vi "CmdGenerate.vi"(1 "Control Value":sgl=1.0 format="%.4f", 2 "Mode":i32=3 format="%x", 3 "Dst":i32=54 format="%x") -> (0 "CMD code":string)   [LabVIEW 2012]
panel:
  out "Revised":u8[](array[numeric]) format="%02x"
  out "Array":u8[](array[numeric]) format="%02x"
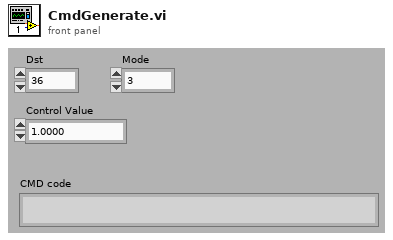
[diagram p1: front panel]
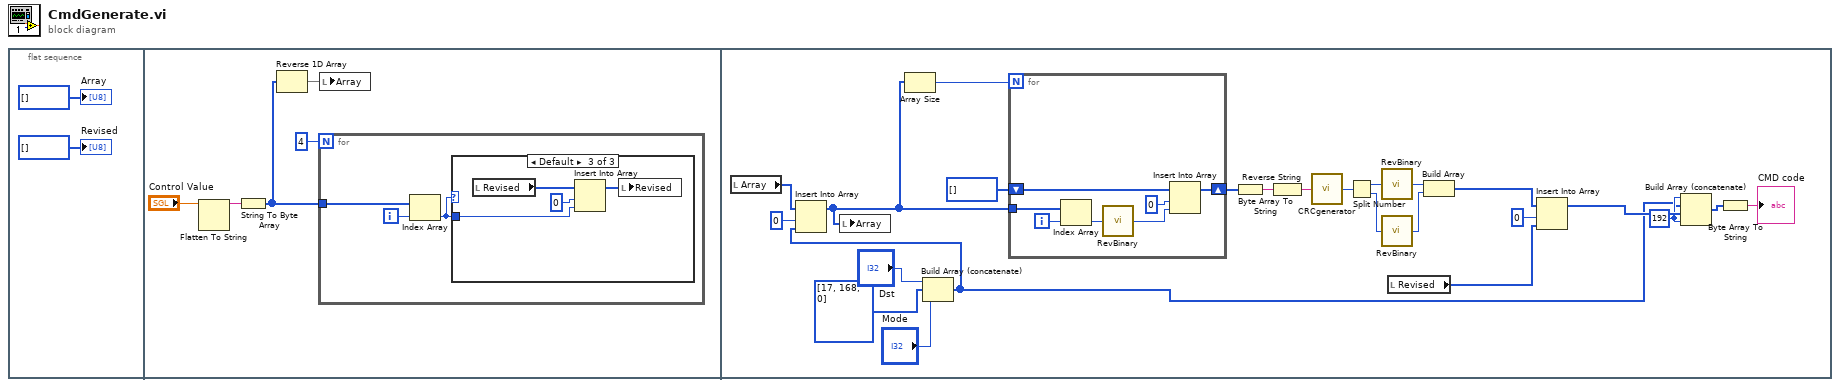
[diagram p0: block diagram]
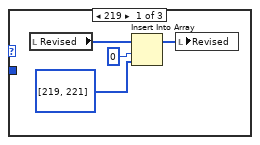
[diagram p2: hidden frame]
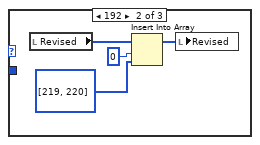
[diagram p3: hidden frame]
diagram:
  n1 = flat-sequence {
    frame #0 {
      "Array" <- u8[] []
      "Revised" <- u8[] []
    }
    frame #1 {
      n2 = Flatten To String(anything="Control Value") -> (data string=w6:string)  [unwired: 3 in, 2 out]
      n3 = String To Byte Array(string=w6) -> (unsigned byte array=w4:u8[])
      n4 = Reverse 1D Array(array=w4) -> (reversed array=w3:u8[])
      n5 = for {
        N: 4 -> [_]
        tunnel: w4 -> [w9]
        i -> [w10]
        n6 = Index Array(array=w9, index=w10) -> (element=w8:u8)
        n7 = case shown="Default" w8 {
          tunnel: w8 -> [_ _ w22]
          frame 219 {
            n8 = local read "Revised"() -> (w11:u8[])
            n9 = Insert Into Array(array=w11, index=0, new element=i32[] [219, 221]) -> (w13:u8[])
            n10 = local write "Revised"(w13) -> ()
          }
          frame 192 {
            n11 = local read "Revised"() -> (w16:u8[])
            n12 = Insert Into Array(array=w16, index=0, new element=i32[] [219, 220]) -> (w15:u8[])
            n13 = local write "Revised"(w15) -> ()
          }
          frame Default {
            n14 = local read "Revised"() -> (w19:u8[])
            n15 = Insert Into Array(array=w19, index=0, new element=w22) -> (w21:u8[])
            n16 = local write "Revised"(w21) -> ()
          }
        }
      }
      n17 = local write "Array"(w3) -> ()
    }
    frame #2 {
      w25 = 192
      n18 = local read "Array"() -> (w46:u8[])
      n19 = Build Array (concatenate)("Dst", i32[] [17, 168, 0], "Mode") -> (w24:i32[])
      n20 = Insert Into Array(array=w46, index=0, new element=w24) -> (w43:u8[])
      n21 = local write "Array"(w43) -> ()
      n22 = Array Size(array=w43) -> (size(s)=w44:i32)
      n23 = for {
        N: w44 -> [_]
        tunnel: w43 -> [w53]
        shift-right: [w50] -> w39
        shift-left: u32[] [] -> [w49]
        i -> [w52]
        n24 = Index Array(array=w53, index=w52) -> (element=w48:u8)
        n25 = call "RevBinary.vi"("Binary"=w48) -> ("Rev Binary"=w47:u32)
        n26 = Insert Into Array(array=w49, index=0, new element=w47) -> (w50:u32[])
      }
      n27 = Byte Array To String(unsigned byte array=w39) -> (string=w40:string)
      n28 = Reverse String(1:w40) -> (0:w41:string)
      n29 = call "CRCgenerator.vi"("String"=w41) -> ("CRC-16-CCITT-0xFFFF"=w38:u16)
      n30 = Split Number(x=w38) -> (hi(x)=w37:u8, lo(x)=w36:u8)
      n31 = call "RevBinary.vi"("Binary"=w37) -> ("Rev Binary"=w33:u32)
      n32 = call "RevBinary.vi"("Binary"=w36) -> ("Rev Binary"=w32:u32)
      n33 = local read "Revised"() -> (w34:u8[])
      n34 = Build Array(w33, w32) -> (w31:u32[])
      n35 = Insert Into Array(array=w31, index=0, new element=w34) -> (w28:u32[])
      n36 = Build Array (concatenate)(w25, w24, w28, w25) -> (w30:u32[])
      n37 = Byte Array To String(unsigned byte array=w30) -> (string=→"CMD code":string)
    }
  }
